vi "EnumDevicesEx2.vi"(5 "nLayerType":u32=1, 11 "error in (no error)":errorcluster caption="错误输入（无错误）") -> (4 "function return":i32, 6 "nDeviceNumReturn":u32, 8 "GigEDeviceArray":T3(array[cluster]), 10 "U3VDeviceArray":T2(array[cluster]), 15 "error out":errorcluster caption="错误输出")   [LabVIEW 2015, in "MvCameraControl.lvlib"]
uses:
  MvCameraControl.lvlib
  MvCameraPatch.dll
panel:
  in  "enSortMethod":T1(ring)
  in  "strManufacturerName":i8[](array[numeric])
  in  "U3VDevice":T4
  in  "GigEDevice":T5
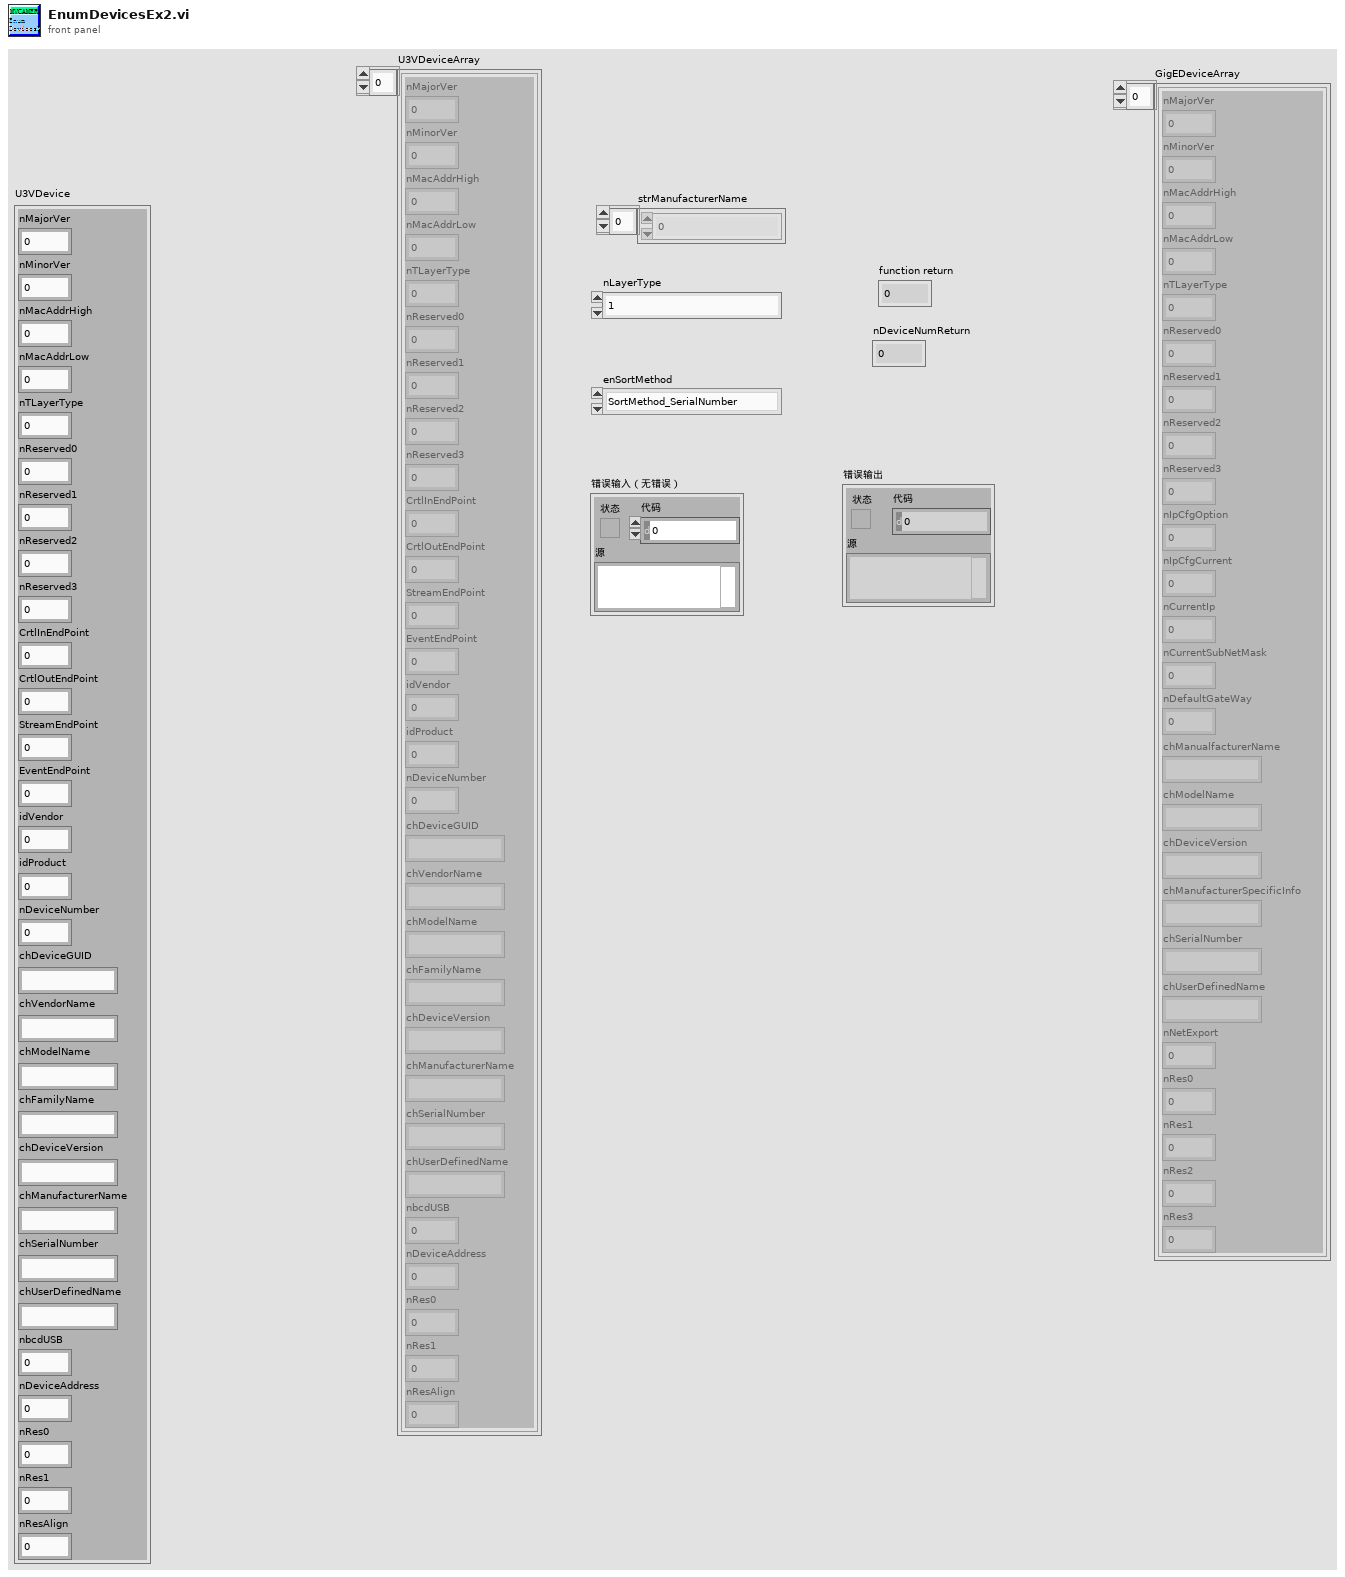
[diagram p1: front panel]
types:
  T1 = enum16{"SortMethod_SerialNumber", "SortMethod_UserID", "SortMethod_CurrentIP_ASC", "SortMethod_CurrentIP_DESC"}
  T2 = cluster{"nMajorVer":u16, "nMinorVer":u16, "nMacAddrHigh":u32, "nMacAddrLow":u32, "nTLayerType":u32, "nReserved0":u32, "nReserved1":u32, "nReserved2":u32, "nReserved3":u32, "CrtlInEndPoint":u8, "CrtlOutEndPoint":u8, "StreamEndPoint":u8, "EventEndPoint":u8, "idVendor":u16, "idProduct":u16, "nDeviceNumber":u32, "chDeviceGUID":string, "chVendorName":string, "chModelName":string, "chFamilyName":string, "chDeviceVersion":string, "chManufacturerName":string, "chSerialNumber":string, "chUserDefinedName":string, "nbcdUSB":u32, "nDeviceAddress":u32, "nRes0":u32, "nRes1":u32, "nResAlign":u32}[]
  T3 = cluster{"nMajorVer":u16, "nMinorVer":u16, "nMacAddrHigh":u32, "nMacAddrLow":u32, "nTLayerType":u32, "nReserved0":u32, "nReserved1":u32, "nReserved2":u32, "nReserved3":u32, "nIpCfgOption":u32, "nIpCfgCurrent":u32, "nCurrentIp":u32, "nCurrentSubNetMask":u32, "nDefaultGateWay":u32, "chManualfacturerName":string, "chModelName":string, "chDeviceVersion":string, "chManufacturerSpecificInfo":string, "chSerialNumber":string, "chUserDefinedName":string, "nNetExport":u32, "nRes0":u32, "nRes1":u32, "nRes2":u32, "nRes3":u32}[]
  T4 = cluster{"nMajorVer":u16, "nMinorVer":u16, "nMacAddrHigh":u32, "nMacAddrLow":u32, "nTLayerType":u32, "nReserved0":u32, "nReserved1":u32, "nReserved2":u32, "nReserved3":u32, "CrtlInEndPoint":u8, "CrtlOutEndPoint":u8, "StreamEndPoint":u8, "EventEndPoint":u8, "idVendor":u16, "idProduct":u16, "nDeviceNumber":u32, "chDeviceGUID":string, "chVendorName":string, "chModelName":string, "chFamilyName":string, "chDeviceVersion":string, "chManufacturerName":string, "chSerialNumber":string, "chUserDefinedName":string, "nbcdUSB":u32, "nDeviceAddress":u32, "nRes0":u32, "nRes1":u32, "nResAlign":u32}
  T5 = cluster{"nMajorVer":u16, "nMinorVer":u16, "nMacAddrHigh":u32, "nMacAddrLow":u32, "nTLayerType":u32, "nReserved0":u32, "nReserved1":u32, "nReserved2":u32, "nReserved3":u32, "nIpCfgOption":u32, "nIpCfgCurrent":u32, "nCurrentIp":u32, "nCurrentSubNetMask":u32, "nDefaultGateWay":u32, "chManualfacturerName":string, "chModelName":string, "chDeviceVersion":string, "chManufacturerSpecificInfo":string, "chSerialNumber":string, "chUserDefinedName":string, "nNetExport":u32, "nRes0":u32, "nRes1":u32, "nRes2":u32, "nRes3":u32}
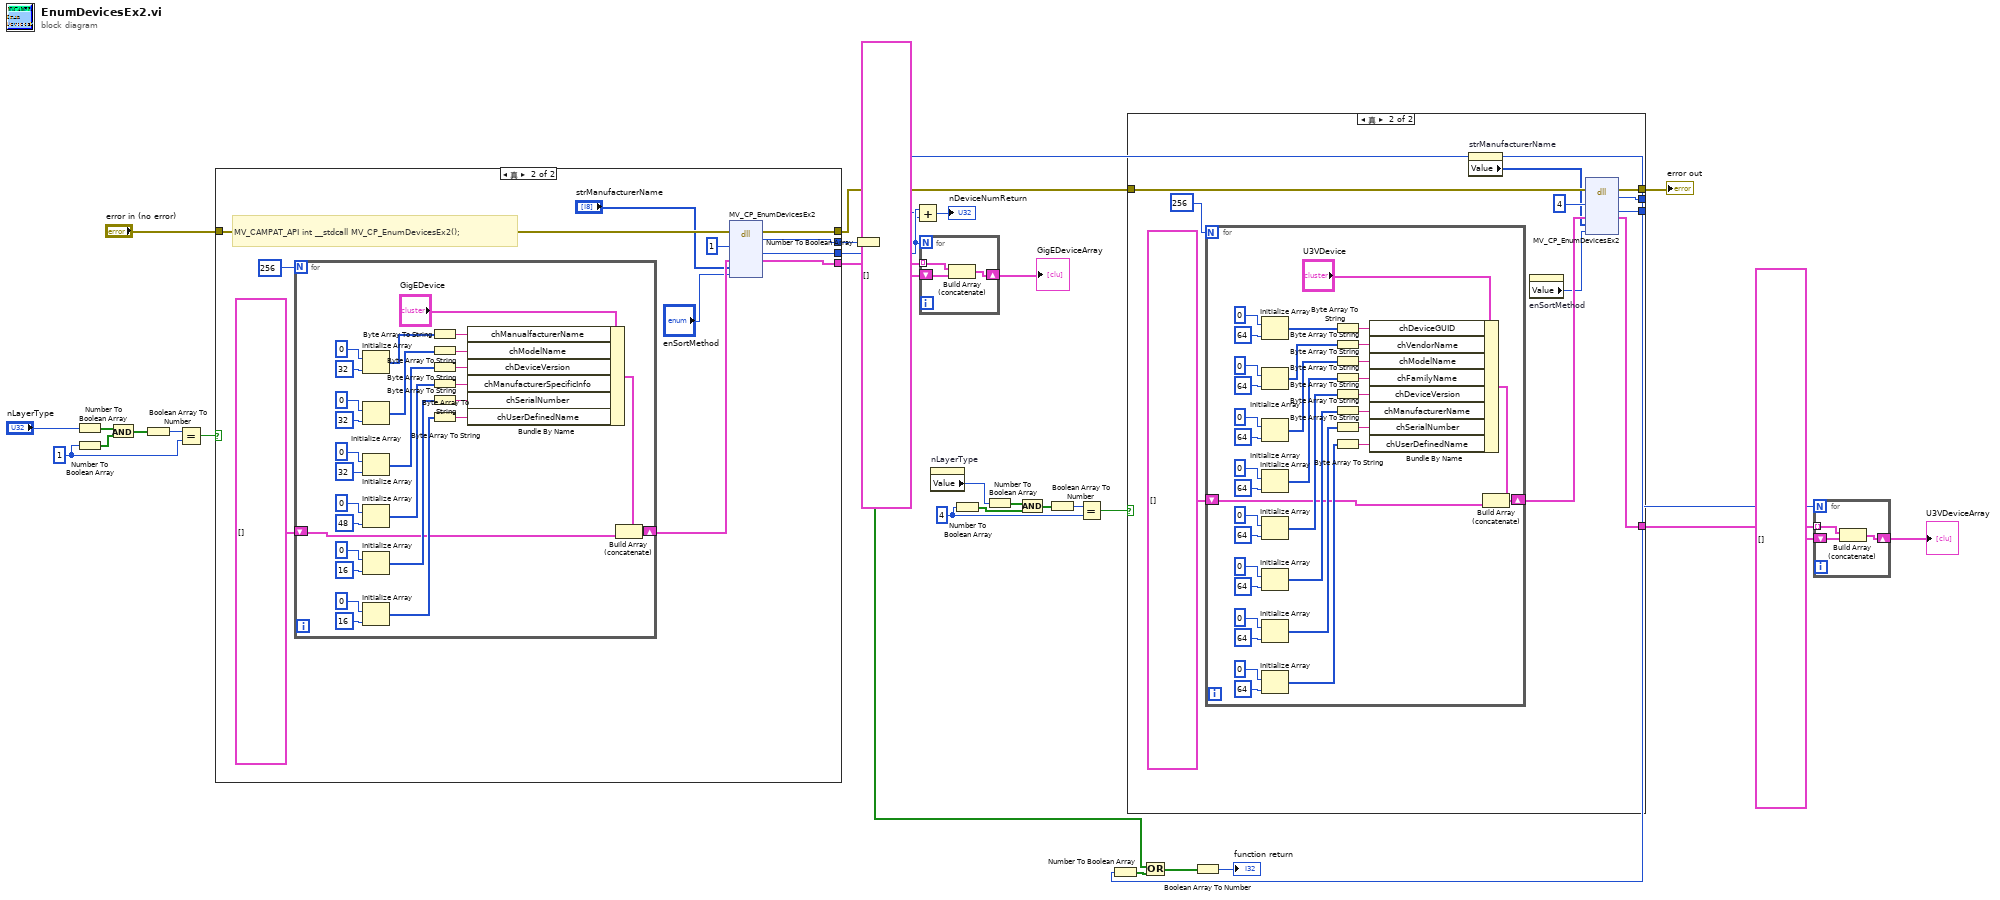
[diagram p0: block diagram]
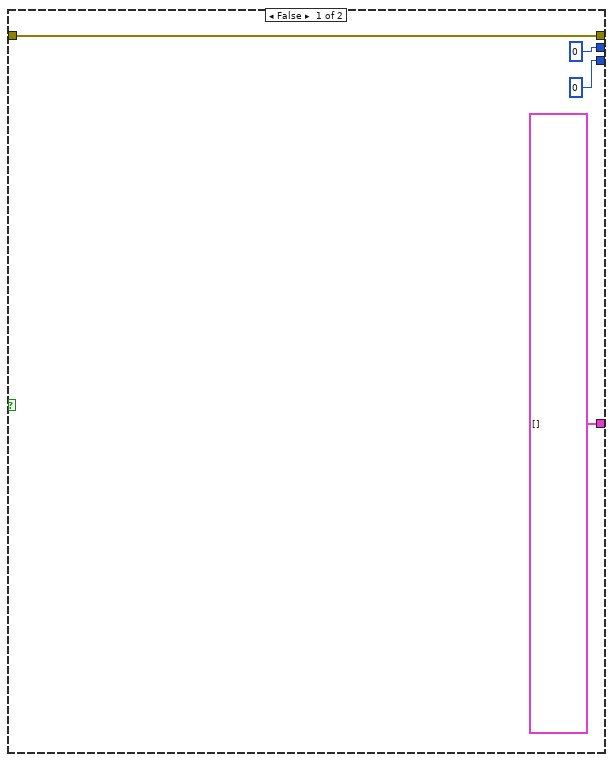
[diagram p2: hidden frame]
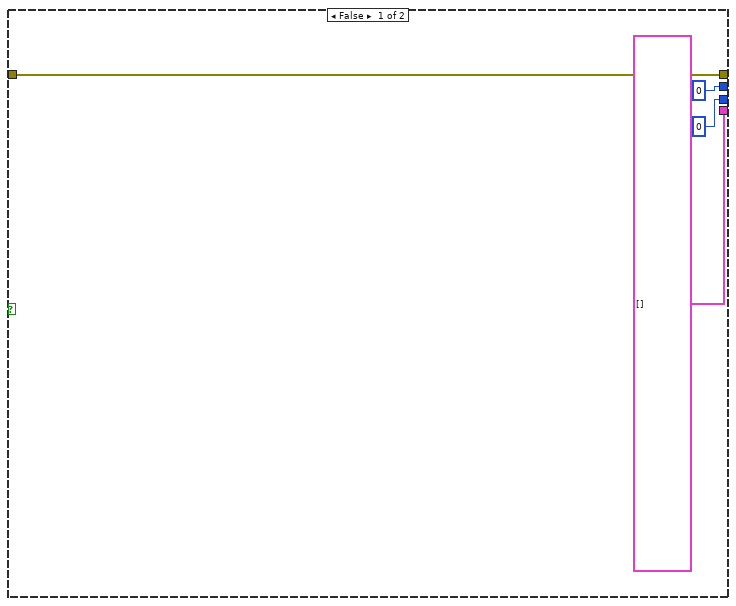
[diagram p3: hidden frame]
diagram:
  w20 = u32 4 ("数字")
  w28 = u32 1 ("数字")
  n1 = Number To Boolean Array(number="nLayerType") -> (Boolean array=w32:bool[])
  n2 = Number To Boolean Array(number=w28) -> (Boolean array=w31:bool[])
  n3 = And(x=w32, y=w31) -> (x .and. y?=w30:bool[])
  n4 = Boolean Array To Number(Boolean array=w30) -> (number=w29:u32)
  n5 = Equal?(x=w29, y=w28) -> (x = y?=w27:bool)
  n6 = case shown="真" w27 {
    tunnel: [0 ("返回类型") w44] -> w16
    tunnel: [u32 0 ("nDeviceNumReturn") w43] -> w9
    tunnel: "error in (no error)" -> [w34 w42]
    tunnel: [w34 w41] -> w11
    tunnel: [T3 [] ("DeviceInfoArray") w39] -> w6
    frame False {
    }
    frame True {
      # "MV_CAMPAT_API int __stdcall MV_CP_EnumDevicesEx2();"
      n7 = for {
        N: 256 -> [_]
        shift-right: [w50] -> w47
        shift-left: T3 [] -> [w48]
        n8 = Initialize Array(u8 0 ("元素"), 32 ("维数大小")) -> (w59:u8[])
        n9 = Initialize Array(u8 0 ("元素"), 32 ("维数大小")) -> (w62:u8[])
        n10 = Initialize Array(u8 0 ("元素"), 32 ("维数大小")) -> (w51:u8[])
        n11 = Initialize Array(u8 0 ("元素"), 48 ("维数大小")) -> (w56:u8[])
        n12 = Initialize Array(u8 0 ("元素"), 16 ("维数大小")) -> (w70:u8[])
        n13 = Initialize Array(u8 0 ("元素"), 16 ("维数大小")) -> (w67:u8[])
        n14 = Byte Array To String(unsigned byte array=w59) -> (string=w71:string)
        n15 = Byte Array To String(unsigned byte array=w62) -> (string=w72:string)
        n16 = Byte Array To String(unsigned byte array=w51) -> (string=w52:string)
        n17 = Byte Array To String(unsigned byte array=w56) -> (string=w73:string)
        n18 = Byte Array To String(unsigned byte array=w70) -> (string=w74:string)
        n19 = Byte Array To String(unsigned byte array=w67) -> (string=w75:string)
        n20 = Bundle By Name(cluster="GigEDevice", "chManualfacturerName"=w71, "chModelName"=w72, "chDeviceVersion"=w52, "chManufacturerSpecificInfo"=w73, "chSerialNumber"=w74, "chUserDefinedName"=w75) -> (w49:T5)
        n21 = Build Array (concatenate)(w49, w48) -> (w50:T3)
      }
      n22 = dll-call lib="MvCameraPatch.dll" fn="MV_CP_EnumDevicesEx2"(error in=w42, "nLayerType"=u32 1, "DeviceInfoArray"=w47, "strManufacturerName"="strManufacturerName", "enSortMethod"="enSortMethod") -> (error out=w41:errorcluster, "返回类型"=w44:i32, "nDeviceNumReturn"=w43:u32, "DeviceInfoArray"=w39:T3)  [unwired: 6 in, 1 out]
    }
  }
  n23 = Number To Boolean Array(number=w16) -> (Boolean array=w15:bool[])
  n24 = for {
    N: w9 -> [_]
    tunnel: w6 -> [w78] mode=indexing
    shift-right: [w76] -> w4
    shift-left: T3 [] -> [w77]
    n25 = Build Array (concatenate)(w78, w77) -> (w76:T3)
  }
  "GigEDeviceArray" <- w4
  n26 = property on="nLayerType" class="DigNum (严格)"() -> ("Value"=w7:u32)  [unwired: 2 in, 2 out]
  n27 = Number To Boolean Array(number=w20) -> (Boolean array=w23:bool[])
  n28 = Number To Boolean Array(number=w7) -> (Boolean array=w24:bool[])
  n29 = And(x=w24, y=w23) -> (x .and. y?=w22:bool[])
  n30 = Boolean Array To Number(Boolean array=w22) -> (number=w21:u32)
  n31 = Equal?(x=w21, y=w20) -> (x = y?=w19:bool)
  n32 = case shown="真" w19 {
    tunnel: [u32 0 ("nDeviceNumReturn") w92] -> w8
    tunnel: [0 ("返回类型") w91] -> w17
    tunnel: w11 -> [w80 w90]
    tunnel: [w80 w89] -> w10
    tunnel: [T2 [] w85] -> w3
    frame False {
    }
    frame True {
      n33 = for {
        N: 256 -> [_]
        shift-right: [w94] -> w87
        shift-left: T2 [] -> [w96]
        n34 = Initialize Array(u8 0 ("元素"), 64 ("维数大小")) -> (w100:u8[])
        n35 = Initialize Array(u8 0 ("元素"), 64 ("维数大小")) -> (w104:u8[])
        n36 = Initialize Array(u8 0 ("元素"), 64 ("维数大小")) -> (w107:u8[])
        n37 = Initialize Array(u8 0 ("元素"), 64 ("维数大小")) -> (w110:u8[])
        n38 = Initialize Array(u8 0 ("元素"), 64 ("维数大小")) -> (w113:u8[])
        n39 = Initialize Array(u8 0 ("元素"), 64 ("维数大小")) -> (w116:u8[])
        n40 = Initialize Array(u8 0 ("元素"), 64 ("维数大小")) -> (w123:u8[])
        n41 = Initialize Array(u8 0 ("元素"), 64 ("维数大小")) -> (w128:u8[])
        n42 = Byte Array To String(unsigned byte array=w100) -> (string=w101:string)
        n43 = Byte Array To String(unsigned byte array=w104) -> (string=w117:string)
        n44 = Byte Array To String(unsigned byte array=w107) -> (string=w118:string)
        n45 = Byte Array To String(unsigned byte array=w110) -> (string=w119:string)
        n46 = Byte Array To String(unsigned byte array=w113) -> (string=w120:string)
        n47 = Byte Array To String(unsigned byte array=w116) -> (string=w124:string)
        n48 = Byte Array To String(unsigned byte array=w123) -> (string=w125:string)
        n49 = Byte Array To String(unsigned byte array=w128) -> (string=w129:string)
        n50 = Bundle By Name(cluster="U3VDevice", "chDeviceGUID"=w101, "chVendorName"=w117, "chModelName"=w118, "chFamilyName"=w119, "chDeviceVersion"=w120, "chManufacturerName"=w124, "chSerialNumber"=w125, "chUserDefinedName"=w129) -> (w95:T4)
        n51 = Build Array (concatenate)(w95, w96) -> (w94:T2)
      }
      n52 = property on="strManufacturerName" class="Arr (严格)"() -> ("Value"=w84:i8[])  [unwired: 2 in, 2 out]
      n53 = property on="enSortMethod" class="Enum (严格)"() -> ("Value"=w83:T1)  [unwired: 2 in, 2 out]
      n54 = dll-call lib="MvCameraPatch.dll" fn="MV_CP_EnumDevicesEx2"(error in=w90, "nLayerType"=u32 4, "DeviceInfoArray"=w87, "strManufacturerName"=w84, "enSortMethod"=w83) -> (error out=w89:errorcluster, "返回类型"=w91:i32, "nDeviceNumReturn"=w92:u32, "DeviceInfoArray"=w85:T2)  [unwired: 6 in, 1 out]
    }
  }
  "error out" <- w10
  n55 = Add(x=w9, y=w8) -> (x+y=→"nDeviceNumReturn":u32)
  n56 = Number To Boolean Array(number=w17) -> (Boolean array=w14:bool[])
  n57 = Or(x=w15, y=w14) -> (x .or. y?=w13:bool[])
  n58 = Boolean Array To Number(Boolean array=w13) -> (number=→"function return":u32)
  n59 = for {
    N: w8 -> [_]
    tunnel: w3 -> [w132] mode=indexing
    shift-right: [w130] -> w1
    shift-left: T2 [] -> [w131]
    n60 = Build Array (concatenate)(w132, w131) -> (w130:T2)
  }
  "U3VDeviceArray" <- w1
